vi "Number To StringValue.vi"(1 "Number In":dbl) -> (0 "String Out":string)   [LabVIEW 2017]
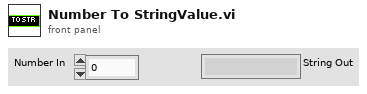
[diagram p1: front panel]
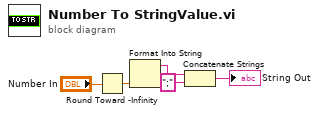
[diagram p0: block diagram]
diagram:
  n1 = Round Toward -Infinity(1:"Number In") -> (0:w1:dbl)
  n2 = Format Into String(w1) -> (resulting string=w5:string)  [unwired: 3 in, 1 out]
  n3 = Concatenate Strings(w5, ";" ("string")) -> (→"String Out":string)
